vi "test take from cube.vi"() -> ()   [LabVIEW 2018]
uses:
  <vilib>/userdefined/High Color/IMAQdx.ctl
  vision/vision info 2.vi
  <vilib>/vision/driver/NI_Vision_Acquisition_Software.lvlib
  <resource>/objmgr/imaqdx.rc
panel:
  in  "angle":i32
  in  "level":i32
  in  "c2":i32
  in  "c1":i32
  in  "stop":bool
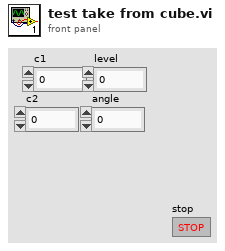
[diagram p1: front panel]
types:
  T1 = typedef "IMAQdx.ctl" = refnum<k21>
  T2 = enum16{"shoulder", "elbow", "wrist", "base", "gripper"}
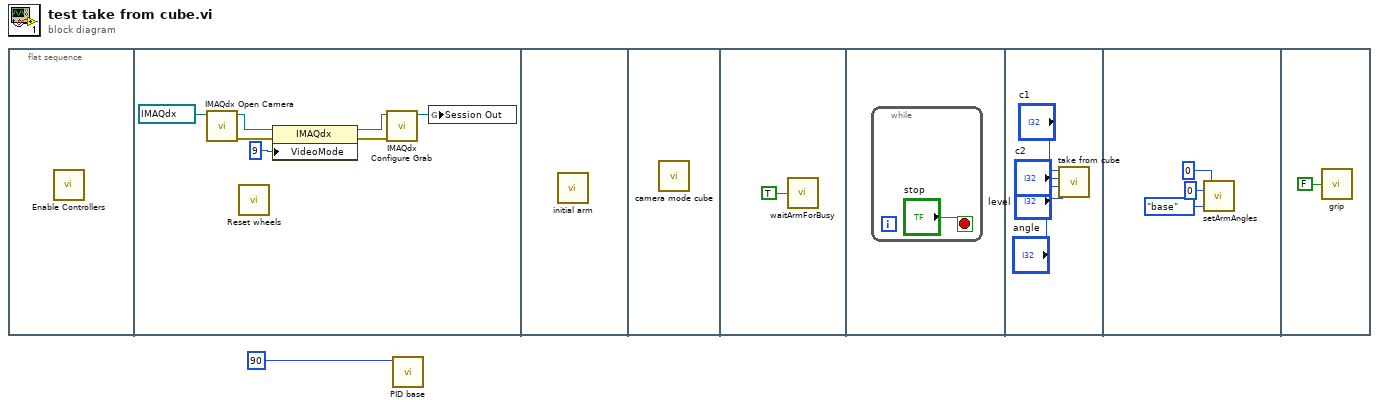
[diagram p0: block diagram]
diagram:
  n1 = flat-sequence {
    frame #0 {
      n2 = call "Enable Controllers.vi"() -> ()  [unwired: 12 in]
    }
    frame #1 {
      n3 = call <vilib>:"IMAQdx Open Camera.vi"("Session In"=T1 "cam0") -> ("error out"=w6:errorcluster, "Session Out"=w5:T1)  [unwired: 9 in]
      n4 = call "Reset wheels.vi"() -> ()  [unwired: 12 in]
      n5 = property class="IMAQdx"(reference=w5, error in=w6, "VideoMode"=u32 9) -> (reference out=w8:T1, error out=w7:errorcluster)
      n6 = call <vilib>:"IMAQdx Configure Grab.vi"("error in"=w7, "Session In"=w8) -> ("Session Out"=w2:T1)  [unwired: 8 in, 1 out]
      n7 = global write "vision info 2.vi" "Session Out"(w2) -> ()
    }
    frame #2 {
      n8 = call "initial arm.vi"() -> ()  [unwired: 12 in]
    }
    frame #3 {
      n9 = call "camera mode cube.vi"() -> ()  [unwired: 12 in]
    }
    frame #4 {
      n10 = call "waitArmForBusy.vi"("base"=TRUE) -> ()
    }
    frame #5 {
      n11 = while {
        stop <- "stop" stop-if-true
      }
    }
    frame #6 {
      n12 = call "take from cube.vi"("level"="level", "angle"="angle", "c2"="c2", "c1"="c1") -> ()  [unwired: 8 in]
    }
    frame #7 {
      n13 = call "setArmAngles.vi"("Enum"=T2."base", "speed"=0, "angle"=0) -> ()  [unwired: 1 in]
    }
    frame #8 {
      n14 = call "grip.vi"("grip"=FALSE) -> ()
    }
  }
  n15 = call "PID base.vi"("base"=90) -> ()  [unwired: 11 in]
